vi "Teleop.vi"(10 "Match Info":T1={"Autonomous Elapsed Seconds"=0.0, "TeleOp Elapsed Seconds"=192.42, "Disabled Elapsed Seconds"=41.06, "Visited Autonomous"=FALSE, "Visited TeleOp"=TRUE, "Visited Disabled"=TRUE, "Autonomous Settings"={"Autonomous Style"=enum."Independent", "VI Refnum"=refnum}}, 11 "Call Context":T2=enum."Stop") -> ()   [LabVIEW 2020]
doc: "This VI is called for each TeleOp packet received from the DS where the robot is not disabled. It is often used to read from the joysticks and update I/O or to update setpoints for timed control loops. It should complete and return within 20 milliseconds or it may miss DS packets."
uses:
  <vilib>/Rock Robotics/WPI/DriverStation/WPI_DriverStationDerivedRobotMode.ctl
  <vilib>/Rock Robotics/WPI/DriverStation/WPI_DriverStationMatch Info.ctl
  Robot Global Data.vi
  <vilib>/Rock Robotics/WPI/Utilities/WPI_GetSetVariantRefNum.vi
  <vilib>/Rock Robotics/Network Tables/NT Write Number.vi
  <vilib>/Rock Robotics/Network Tables/NT Write Numeric Array.vi
  <vilib>/Rock Robotics/Network Tables/NT Write Boolean.vi
panel:
  in  "Drive":bool
  in  "DriveScale":dbl(slide)=0.7556179775280899 min=0.25 max=1.0 step=0.1 scale=0.25..1.0
  in  "Steering Scale":dbl(slide)=0.6418539325842696 min=0.25 max=1.0 step=0.1 scale=0.25..1.0
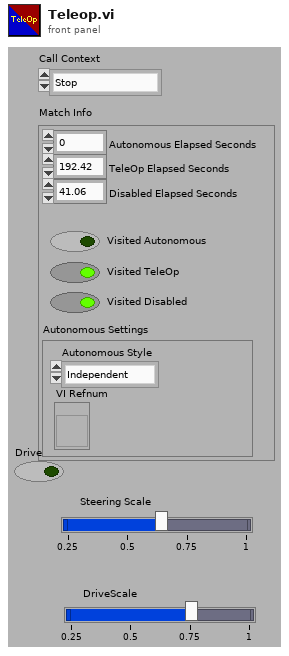
[diagram p1: front panel]
types:
  T1 = typedef "WPI_DriverStationMatch Info.ctl" = cluster{"Autonomous Elapsed Seconds":dbl, "TeleOp Elapsed Seconds":dbl, "Disabled Elapsed Seconds":dbl, "Visited Autonomous":bool, "Visited TeleOp":bool, "Visited Disabled":bool, "Autonomous Settings":cluster{"Autonomous Style":enum16{"Iterative", "Independent"}, "VI Refnum":refnum<vi>}}
  T2 = typedef "WPI_DriverStationDerivedRobotMode.ctl" = enum16{"Init", "Execute", "Stop"}
  T3 = typedef "WPI_RobotDriveDevRef.ctl" = cluster{"DevStatus":errorcluster, "Motors[]":T4[], "Square Inputs":bool, "Max Output":dbl}
  T4 = typedef "WPI_MotorControlDeviceRef.ctl" = cluster{"DeviceStatus":errorcluster, "Type":T5, "PWM":cluster{"PWM Channel":T6, "DeadBand":T7}, "CAN":cluster{"Device Number":u8, "SetOutput VI Ref":variant, "GetOutput VI Ref":variant, "Enable VI Ref":variant, "Disable VI Ref":variant, "Data":variant}, "Invert":bool, "DIO PWM":cluster{"PWM \"Enable\" Channel":T6, "DIOChannel":T8, "PWM Rate":dbl}}
  T5 = typedef "WPI_MotorControlType.ctl" = enum16{"PWM", "CAN", "DIO PWM"}
  T6 = typedef "FPGA_DIOPWMChannel.ctl" = enum8{"PWM 0", "PWM 1", "PWM 2", "PWM 3", "PWM 4", "PWM 5", "PWM 6", "PWM 7", "PWM 8", "PWM 9", "PWM MXP 0", "PWM MXP 1", "PWM MXP 2", "PWM MXP 3", "PWM MXP 4", "PWM MXP 5", "PWM MXP 6", "PWM MXP 7", "PWM MXP 8", "PWM MXP 9", "Invalid"}
  T7 = typedef "WPI_PWMDeadband.ctl" = cluster{"Name":string, "maxPositivePwm":i32, "minPositivePwm":i32, "centerPwm":i32, "maxNegativePwm":i32, "minNegativePwm":i32, "angularRange":u16}
  T8 = typedef "FPGA_DIOChannel.ctl" = enum8{"DIO 0", "DIO 1", "DIO 2", "DIO 3", "DIO 4", "DIO 5", "DIO 6", "DIO 7", "DIO 8", "DIO 9", "DIO MXP 0", "DIO MXP 1", "DIO MXP 2", "DIO MXP 3", "DIO MXP 4", "DIO MXP 5", "DIO MXP 6", "DIO MXP 7", "DIO MXP 8", "DIO MXP 9", "DIO MXP 10", "DIO MXP 11", "DIO MXP 12", "DIO MXP 13", "DIO MXP 14", "DIO MXP 15", "SPI Port CS1", "SPI Port CS2", "SPI Port CS3", "SPI Port MISO", "SPI Port MOSI", "Invalid"}
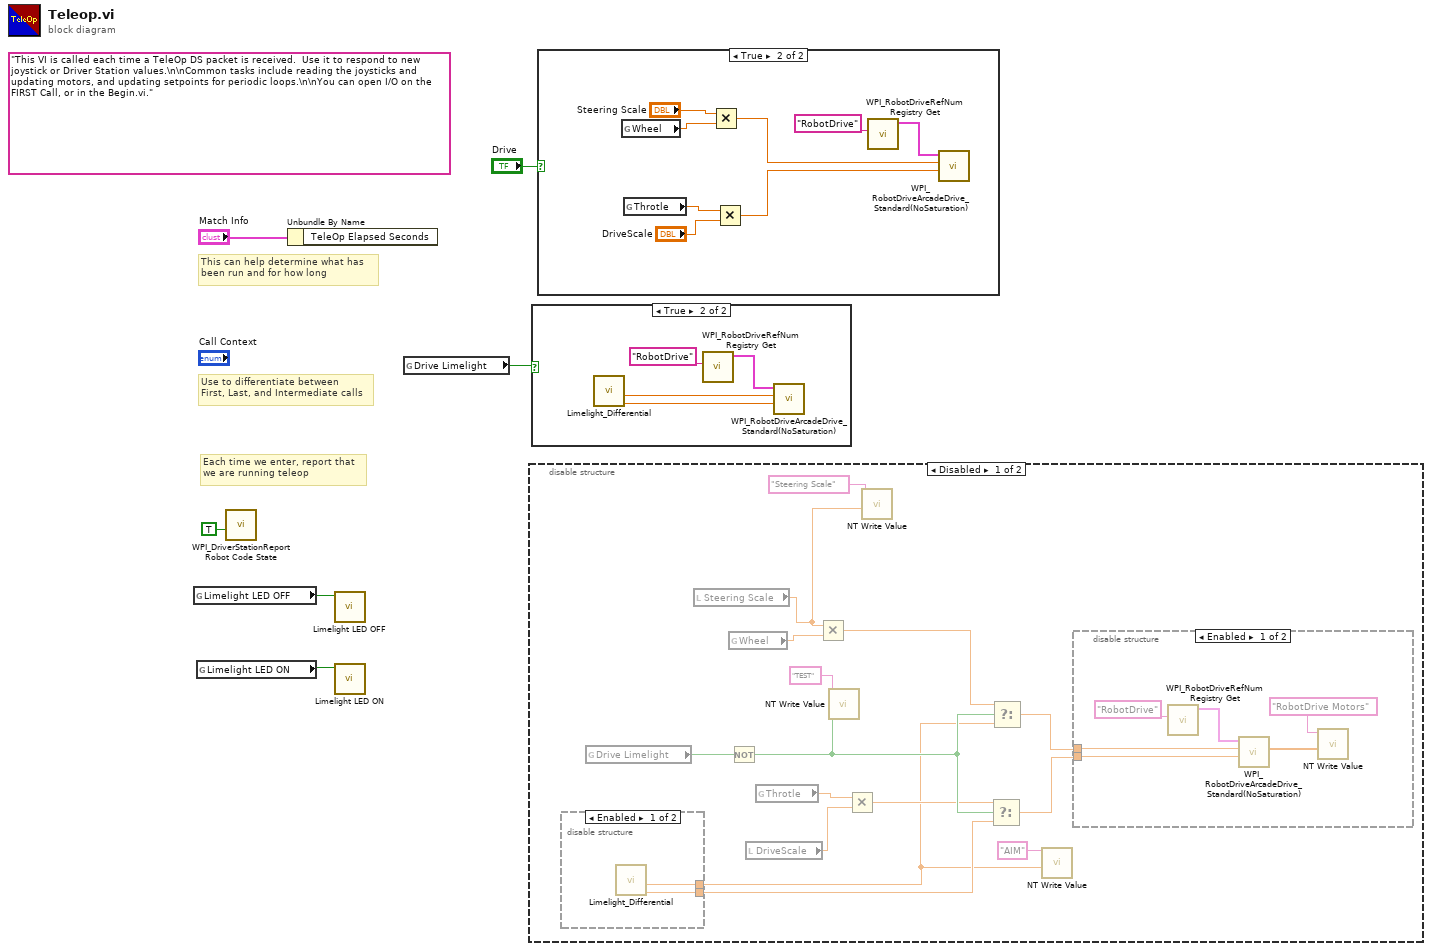
[diagram p0: block diagram]
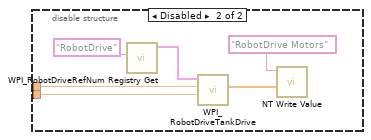
[diagram p4: hidden frame]
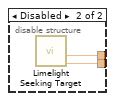
[diagram p5: hidden frame]
diagram:
  (unwired) "This VI is called each time a TeleOp DS packet is received.  Use it to respond to new joystick or Driver Station values.\n\nCommon tasks include reading the joysticks and updating motors, and updating setpoints for periodic loops.\n\nYou can open I/O on the FIRST Call, or in the Begin.vi."
  # "Each time we enter, report that\nwe are running teleop"
  # "Use to differentiate between\nFirst, Last, and Intermediate calls"
  # "This can help determine what has\nbeen run and for how long"
  n1 = global read "Robot Global Data.vi" "Limelight LED OFF"() -> (w3:bool)
  n2 = global read "Robot Global Data.vi" "Limelight LED ON"() -> (w4:bool)
  n3 = call <vilib>:"WPI_DriverStationReport Robot Code State.vi"("TeleOp"=TRUE ("Autonomous")) -> ()  [unwired: 10 in, 1 out]
  n4 = Unbundle By Name("Match Info") -> ()  [unwired: 1 out]
  n5 = call "Limelight LED OFF.vi"("LED OFF (T)"=w3) -> ()  [unwired: 11 in]
  n6 = call "Limelight LED ON.vi"("D Start  9"=w4) -> ()  [unwired: 10 in, 1 out]
  n7 = global read "Robot Global Data.vi" "Drive Limelight"() -> (w1:bool)
  n8 = disable-structure shown="Disabled" {
    frame Disabled {
      n9 = disable-structure shown="Enabled" {
        disable-tunnel: [w35 w36] -> w13
        disable-tunnel: [w34 w37] -> w12
        frame Enabled {
          n10 = call "Limelight_Differential.vi"() -> ("DriveCommand"=w35:dbl, "SteerCommand"=w34:dbl)  [unwired: 8 in, 1 out]
        }
        frame Disabled {
          n11 = call "Limelight Seeking Target.vi"() -> ("DriveCommand"=w36:dbl, "SteerCommand"=w37:dbl)  [unwired: 8 in, 1 out]
        }
      }
      n12 = global read "Robot Global Data.vi" "Drive Limelight"() -> (w9:bool)
      n13 = local read "Steering Scale"() -> (w7:dbl)
      n14 = global read "Robot Global Data.vi" "Wheel"() -> (w10:dbl)
      n15 = Not(x=w9) -> (.not. x?=w17:bool)
      n16 = local read "DriveScale"() -> (w8:dbl)
      n17 = global read "Robot Global Data.vi" "Throtle"() -> (w11:dbl)
      n18 = Multiply(x=w7, y=w10) -> (x*y=w16:dbl)
      n19 = call-poly <vilib>:"NT Write Value.vi"("Boolean"=w17, "Name"="TEST") -> ()  [unwired: 9 in, 1 out]
      n20 = Multiply(x=w11, y=w8) -> (x*y=w15:dbl)
      n21 = call-poly <vilib>:"NT Write Value.vi"("Numeric"=w7, "Name"="Steering Scale") -> ()  [unwired: 9 in, 1 out]
      n22 = Select(t=w15, s=w17, f=w13) -> (s? t:f=w20:dbl)
      n23 = Select(t=w16, s=w17, f=w12) -> (s? t:f=w21:dbl)
      n24 = call-poly <vilib>:"NT Write Value.vi"("Numeric"=w12, "Name"="AIM") -> ()  [unwired: 9 in, 1 out]
      n25 = disable-structure shown="Enabled" {
        disable-tunnel: w21 -> [w23 w29]
        disable-tunnel: w20 -> [w22 w28]
        frame Enabled {
          n26 = call <vilib>:"WPI_RobotDriveRefNum Registry Get.vi"("refnum name"="RobotDrive") -> ("RobotDriveDevRef"=w26:T3)  [unwired: 1 in, 9 out]
          n27 = call <vilib>:"WPI_RobotDriveArcadeDrive_Standard(NoSaturation).vi"("Y axis value"=w22, "X axis value"=w23, "RobotDriveDevRef"=w26) -> ("Motor Values"=w25:dbl[])  [unwired: 1 in, 7 out]
          n28 = call-poly <vilib>:"NT Write Value.vi"("Numeric Array"=w25, "Name"="RobotDrive Motors") -> ()  [unwired: 9 in, 1 out]
        }
        frame Disabled {
          n29 = call <vilib>:"WPI_RobotDriveRefNum Registry Get.vi"("refnum name"="RobotDrive") -> ("RobotDriveDevRef"=w32:T3)  [unwired: 1 in, 9 out]
          n30 = call <vilib>:"WPI_RobotDriveTankDrive.vi"("Right axis value"=w28, "Left axis value"=w29, "RobotDriveDevRef"=w32) -> ("Motor Values"=w31:dbl[])  [unwired: 6 in, 2 out]
          n31 = call-poly <vilib>:"NT Write Value.vi"("Numeric Array"=w31, "Name"="RobotDrive Motors") -> ()  [unwired: 9 in, 1 out]
        }
      }
    }
    frame Enabled {
    }
  }
  n32 = case shown="True" w1 {
    frame False {
    }
    frame True {
      n33 = call "Limelight_Differential.vi"() -> ("DriveCommand"=w41:dbl, "SteerCommand"=w40:dbl)  [unwired: 8 in, 1 out]
      n34 = call <vilib>:"WPI_RobotDriveRefNum Registry Get.vi"("refnum name"="RobotDrive") -> ("RobotDriveDevRef"=w38:T3)  [unwired: 1 in, 9 out]
      n35 = call <vilib>:"WPI_RobotDriveArcadeDrive_Standard(NoSaturation).vi"("Y axis value"=w41, "X axis value"=w40, "RobotDriveDevRef"=w38) -> ()  [unwired: 1 in, 8 out]
    }
  }
  n36 = case shown="True" "Drive" {
    frame False {
    }
    frame True {
      n37 = global read "Robot Global Data.vi" "Wheel"() -> (w44:dbl)
      n38 = global read "Robot Global Data.vi" "Throtle"() -> (w45:dbl)
      n39 = Multiply(x="Steering Scale", y=w44) -> (x*y=w49:dbl)
      n40 = Multiply(x=w45, y="DriveScale") -> (x*y=w47:dbl)
      n41 = call <vilib>:"WPI_RobotDriveRefNum Registry Get.vi"("refnum name"="RobotDrive") -> ("RobotDriveDevRef"=w42:T3)  [unwired: 1 in, 9 out]
      n42 = call <vilib>:"WPI_RobotDriveArcadeDrive_Standard(NoSaturation).vi"("Y axis value"=w47, "X axis value"=w49, "RobotDriveDevRef"=w42) -> ()  [unwired: 1 in, 8 out]
    }
  }
